vi "get channels.vi"(11 "module configuration in":refnum<class "Binary datalogger configuration.lvclass">) -> (2 "channels":refnum<class "TBM channel.lvclass">[](array[class]), 3 "module configuration out":refnum<class "Binary datalogger configuration.lvclass">)   [LabVIEW 2013, in "Binary datalogger configuration.lvclass"]
uses:
  Binary datalogger configuration.lvclass
  <vilib>/NI/Tag Bus Module Framework/channel/TBM channel.lvclass
  Binary datalogger configuration.lvclass/Binary datalogger configuration.ctl
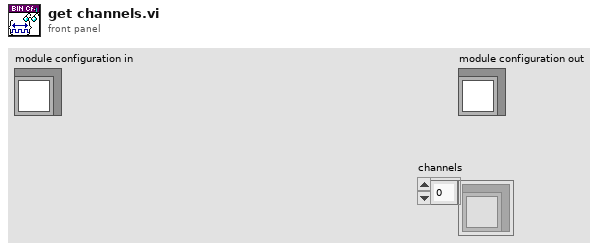
[diagram p1: front panel]
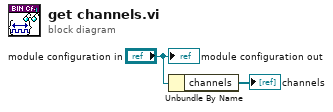
[diagram p0: block diagram]
diagram:
  n1 = Unbundle By Name("module configuration in") -> ("channels"=→"channels":refnum<class "TBM channel.lvclass">[])
  "module configuration out" <- "module configuration in"
